vi "Cfg Notifier.vi"(7 "State":T1=enum."Get", 11 "Data In":string) -> (0 "error out":errorcluster, 2 "timed out?":bool, 3 "Data Out":string)   [LabVIEW 2014]
doc: "This VI facillitates communication between the web services and the controller. This VI stores a notifier that is used to ship configuration data from the controller to the web services. The configuration notifier might be used at startup and whenever the controller may update the current state of controls (such as when the resonant frequency changes or if a calibration is running)."
uses:
  Controls/Notifier Enum.ctl
  Controller.lvclass
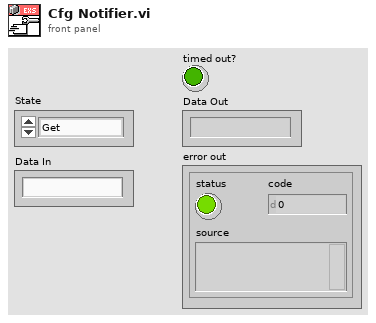
[diagram p1: front panel]
types:
  T1 = typedef "Controller.lvlib/Controller.lvclass/Notifier Enum.ctl" = enum16{"Initialize", "Get", "Set", "Close"}
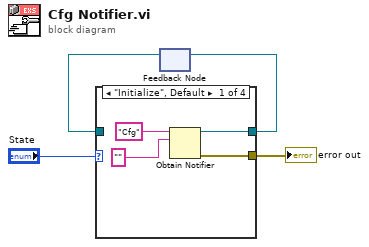
[diagram p0: block diagram]
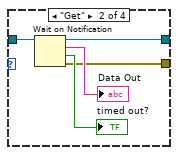
[diagram p2: hidden frame]
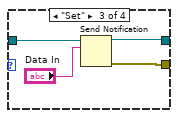
[diagram p3: hidden frame]
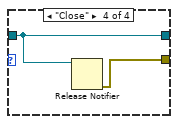
[diagram p4: hidden frame]
diagram:
  n1 = feedback #1() -> (w3:refnum<notifier>)  [unwired: 1 in]
  n2 = case shown="\"Initialize\", Default" "State" {
    tunnel: [w6 w10 w16 w18] -> w4
    tunnel: w3 -> [_ w13 w17 w18]
    tunnel: [w5 w9 w15 w19] -> w2
    frame "Initialize", Default {
      n3 = Obtain Notifier(name (unnamed)="Cfg", notification data type="" ("name (unnamed)")) -> (notifier out=w6:refnum<notifier>, error out=w5:errorcluster)  [unwired: 2 in, 1 out]
    }
    frame "Get" {
      n4 = Wait on Notification(notifier=w13) -> (notifier out=w10:refnum<notifier>, notification=→"Data Out":string, timed out?=→"timed out?":bool, error out=w9:errorcluster)  [unwired: 3 in]
    }
    frame "Set" {
      n5 = Send Notification(notification="Data In", notifier=w17) -> (notifier out=w16:refnum<notifier>, error out=w15:errorcluster)  [unwired: 1 in]
    }
    frame "Close" {
      n6 = Release Notifier(notifier=w18) -> (error out=w19:errorcluster)  [unwired: 2 in, 2 out]
    }
  }
  "error out" <- w2
  n7 = feedback-in #1(w4) -> ()
